vi "Instrument_Detection.vi"(8 "error in (no error)":errorcluster, 10 "GPIB Address":u32) -> (0 "error IO":errorcluster, 2 "ID":string, 5 "Instrument detected?":bool[](array[boolean]))   [LabVIEW 2020]
uses:
  <vilib>/Utility/error.llb/DialogType.ctl
panel:
  in  "?":errorcluster
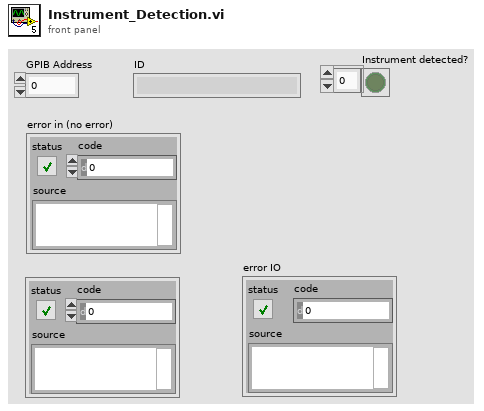
[diagram p1: front panel]
types:
  T1 = typedef "DialogType.ctl" = u16
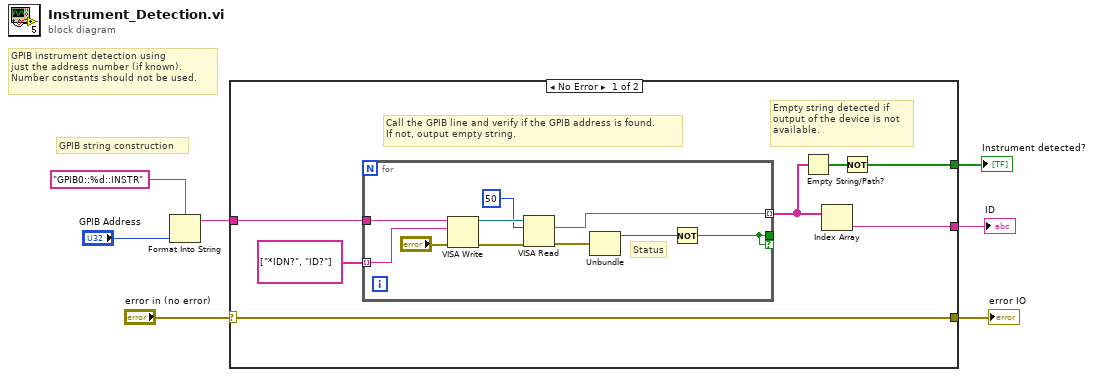
[diagram p0: block diagram]
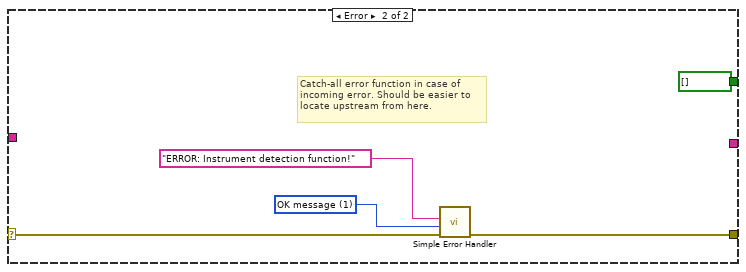
[diagram p2: hidden frame]
diagram:
  # "GPIB string construction"
  # "GPIB instrument detection using\njust the address number (if known).\nNumber constants should not be used."
  n1 = Format Into String(format string="GPIB0::%d::INSTR" ("initial string"), "GPIB Address") -> (resulting string=w5:string)  [unwired: 2 in, 1 out]
  n2 = case shown="No Error" "error in (no error)" {
    selector: "error in (no error)" -> [w12 w29]
    tunnel: w5 -> [w14 _]
    tunnel: [w12 w27] -> w3
    tunnel: [w11 _] -> w2
    tunnel: [w8 bool[] []] -> w1
    frame No Error {
      # "Empty string detected if\noutput of the device is not\navailable."
      # "Call the GPIB line and verify if the GPIB address is found.\nIf not, output empty string."
      n3 = for {
        tunnel: w14 -> [w24]
        tunnel: string[] ["*IDN?", "ID?"] -> [w23] mode=indexing
        tunnel: [w16] -> w10 mode=indexing
        tunnel: [w15] -> _ if=w15
        # "Status"
        n4 = VISA Write(VISA resource name=w24, write buffer=w23, error in (no error)="?") -> (VISA resource name out=w21:refnum<visa-resource-name>, error out=w22:errorcluster)  [unwired: 1 out]
        n5 = VISA Read(VISA resource name=w21, byte count=u32 50, error in (no error)=w22) -> (read buffer=w16:string, error out=w18:errorcluster)  [unwired: 2 out]
        n6 = Unbundle(w18) -> ("status"=w17:bool)  [unwired: 2 out]
        n7 = Not(x=w17) -> (.not. x?=w15:bool)
      }
      n8 = Empty String/Path?(string/path=w10) -> (empty?=w9:bool[])
      n9 = Index Array(array=w10) -> (element=w11:string)  [unwired: 1 in]
      n10 = Not(x=w9) -> (.not. x?=w8:bool[])
    }
    frame Error {
      w28 = T1 1 items=["no dialog", "OK message", "continue or stop message", "OK message + warnings", "continue/stop + warnings"] ("type of dialog (OK msg:1)")
      # "Catch-all error function in case of\nincoming error. Should be easier to\nlocate upstream from here."
      n11 = call <vilib>:"Simple Error Handler.vi"("error source (\" \")"="ERROR: Instrument detection function!" ("error source (\" \")"), "type of dialog (OK msg:1)"=w28, "error in (no error)"=w29) -> ("error out"=w27:errorcluster)  [unwired: 2 in, 4 out]
    }
  }
  "error IO" <- w3
  "ID" <- w2
  "Instrument detected?" <- w1
